vi "Keyence.Cmd.OperationCommands.Get.vi"(6 "Timeout [ms] (1000)":i32=1000, 8 "error in":errorcluster, 10 "Cmd":T1, 11 "cID in":refnum<k5>) -> (0 "error out":errorcluster, 1 "OK?":bool, 2 "Response":string, 3 "cID out":refnum<k5>)   [LabVIEW 2015]
uses:
  Keyence.Cmd.OperationCommands.ctl
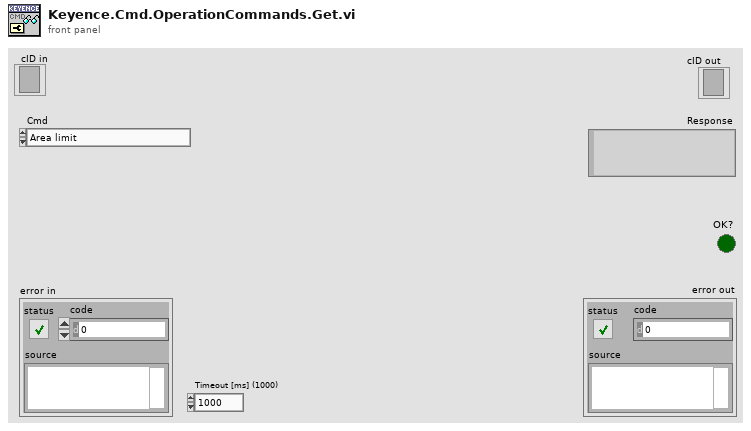
[diagram p1: front panel]
types:
  T1 = typedef "Keyence.Cmd.OperationCommands.ctl" = enum16{"Area limit"}
  T2 = enum16{"Standard", "Buffered", "CRLF", "Immediate"}
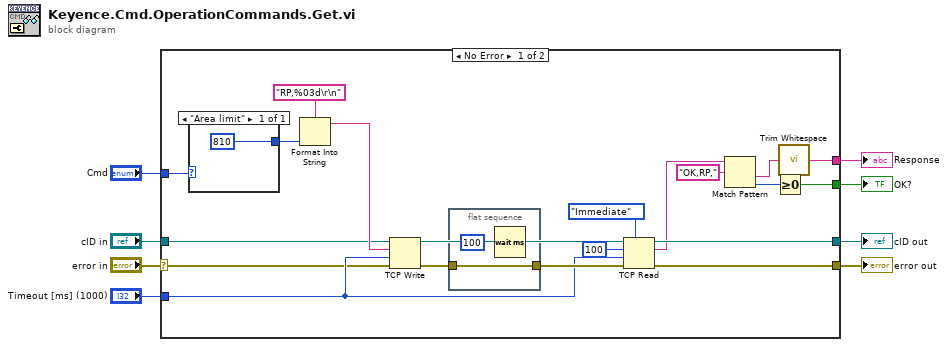
[diagram p0: block diagram]
diagram:
  n1 = case shown="No Error" "error in" {
    selector: "error in" -> [w20 w32]
    tunnel: "Timeout [ms] (1000)" -> [w22 _]
    tunnel: "Cmd" -> [w26 _]
    tunnel: "cID in" -> [w21 w33]
    tunnel: [w12 w33] -> w4
    tunnel: [w13 w32] -> w1
    tunnel: [w9 _] -> w3
    tunnel: [w14 _] -> w2
    frame No Error {
      n2 = case shown="\"Area limit\"" w26 {
        tunnel: [810] -> w15
        frame "Area limit" {
        }
      }
      n3 = Format Into String(format string="RP,%03d\r\n", w15) -> (resulting string=w25:string)  [unwired: 2 in, 1 out]
      n4 = TCP Write(connection ID=w21, data in=w25, error in (no error)=w20, 9:w22) -> (connection ID out=w23:refnum<k5>, error out=w28:errorcluster)  [unwired: 1 out]
      n5 = flat-sequence {
        tunnel: w28 -> [w31]
        tunnel: [w31] -> w24
        frame #0 {
          n6 = Wait (ms)(milliseconds to wait=u32 100) -> ()  [unwired: 1 out]
        }
      }
      n7 = TCP Read(connection ID=w23, bytes to read=100, error in (no error)=w24, 7:T2."Immediate" ("mode (standard)"), 9:w22) -> (connection ID out=w12:refnum<k5>, data out=w11:string, error out=w13:errorcluster)
      n8 = Match Pattern(string=w11, regular expression="OK,RP,") -> (after substring=w10:string, offset past match=w16:i32)  [unwired: 1 in, 2 out]
      n9 = Greater Or Equal To 0?(x=w16) -> (x >= 0?=w14:bool)
      n10 = call <vilib>:"Trim Whitespace.vi"("string"=w10) -> ("trimmed string"=w9:string)  [unwired: 1 in]
    }
    frame Error {
    }
  }
  "cID out" <- w4
  "Response" <- w3
  "OK?" <- w2
  "error out" <- w1
